vi "Faults and Position data.vi"(8 "error in (no error)":errorcluster, 11 "Controller In":refnum<k24>) -> (0 "error out":errorcluster, 1 "Positions":dbl[](array[numeric]), 2 "Faults":string[](array[string]), 3 "Controller Out":refnum<k24>)   [LabVIEW 2011]
uses:
  C:/Users/Admin/Desktop/Gantry Code Transfer/source/Code Transfer/Aerotech.A3200.dll
  Aerotech.A3200.dll
  AxisDiagPacket.ctl
panel:
  out "Axes":T1[](array[typedef])
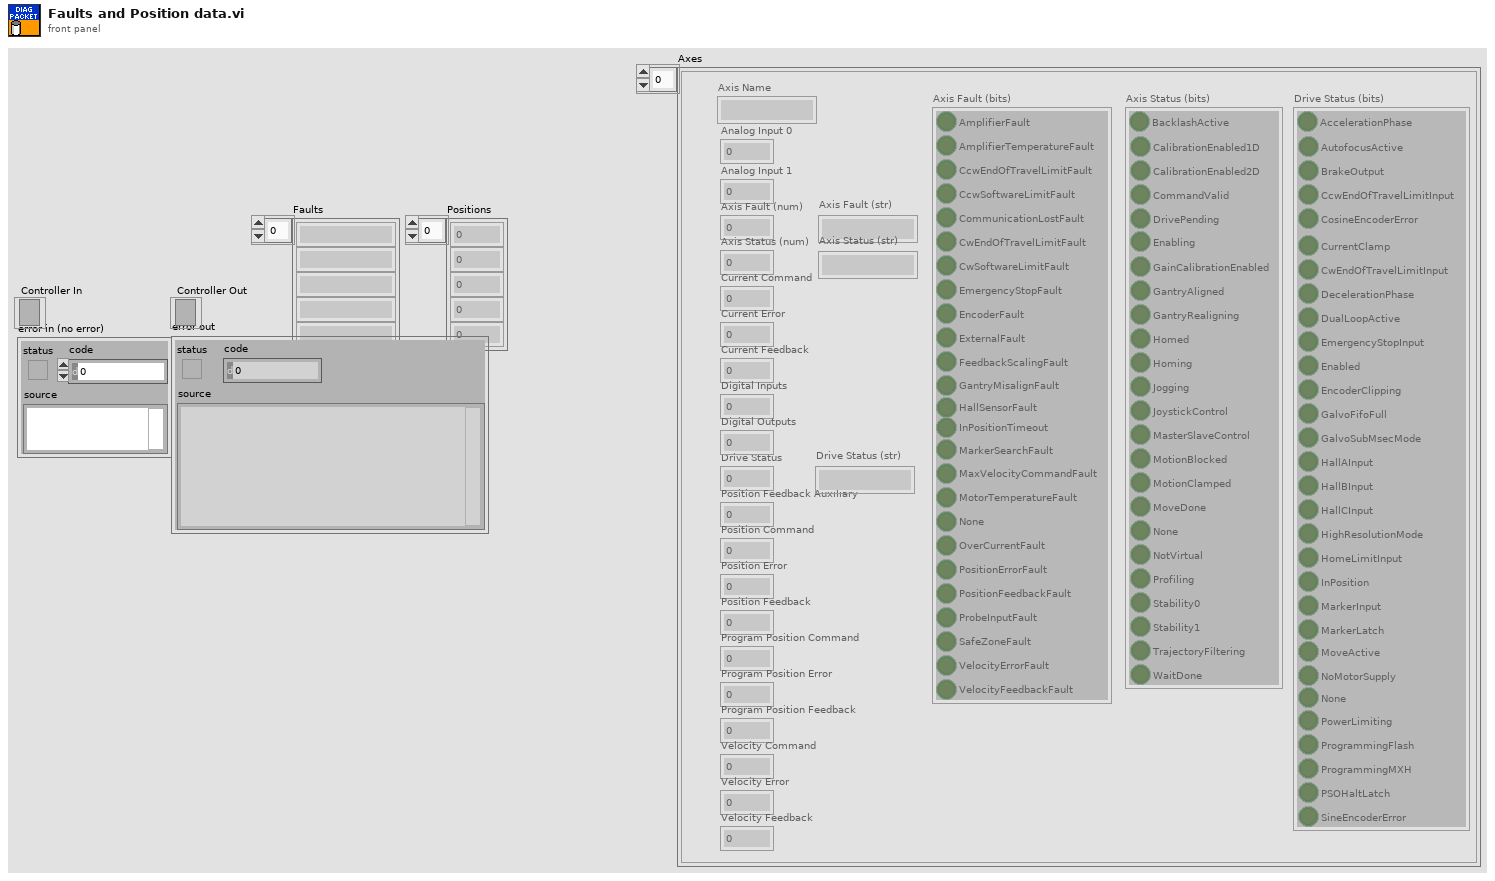
[diagram p1: front panel]
types:
  T1 = typedef "AxisDiagPacket.ctl" = cluster{"Axis Name":string, "Analog Input 0":dbl, "Analog Input 1":dbl, "Axis Fault (num)":i32, "Axis Fault (str)":string, "Axis Fault (bits)":cluster{"AmplifierFault":bool, "AmplifierTemperatureFault":bool, "CcwEndOfTravelLimitFault":bool, "CcwSoftwareLimitFault":bool, "CommunicationLostFault":bool, "CwEndOfTravelLimitFault":bool, "CwSoftwareLimitFault":bool, "EmergencyStopFault":bool, "EncoderFault":bool, "ExternalFault":bool, "FeedbackScalingFault":bool, "GantryMisalignFault ":bool, "HallSensorFault":bool, "InPositionTimeout":bool, "MarkerSearchFault":bool, "MaxVelocityCommandFault":bool, "MotorTemperatureFault":bool, "None":bool, "OverCurrentFault":bool, "PositionErrorFault":bool, "PositionFeedbackFault":bool, "ProbeInputFault":bool, "SafeZoneFault":bool, "VelocityErrorFault":bool, "VelocityFeedbackFault":bool}, "Axis Status (num)":i32, "Axis Status (str)":string, "Axis Status (bits)":cluster{"BacklashActive":bool, "CalibrationEnabled1D":bool, "CalibrationEnabled2D":bool, "CommandValid":bool, "DrivePending":bool, "Enabling":bool, "GainCalibrationEnabled":bool, "GantryAligned":bool, "GantryRealigning":bool, "Homed":bool, "Homing":bool, "Jogging":bool, "JoystickControl":bool, "MasterSlaveControl":bool, "MotionBlocked":bool, "MotionClamped":bool, "MoveDone":bool, "None":bool, "NotVirtual":bool, "Profiling":bool, "Stability0":bool, "Stability1":bool, "TrajectoryFiltering":bool, "WaitDone":bool}, "Current Command":sgl, "Current Error":sgl, "Current Feedback":sgl, "Digital Inputs":i32, "Digital Outputs":i32, "Drive Status":i32, "Drive Status (str)":string, "Drive Status (bits)":cluster{"AccelerationPhase":bool, "AutofocusActive":bool, "BrakeOutput":bool, "CcwEndOfTravelLimitInput":bool, "CosineEncoderError":bool, "CurrentClamp":bool, "CwEndOfTravelLimitInput":bool, "DecelerationPhase":bool, "DualLoopActive":bool, "EmergencyStopInput":bool, "Enabled":bool, "EncoderClipping":bool, "GalvoFifoFull":bool, "GalvoSubMsecMode":bool, "HallAInput":bool, "HallBInput":bool, "HallCInput":bool, "HighResolutionMode":bool, "HomeLimitInput":bool, "InPosition":bool, "MarkerInput":bool, "MarkerLatch":bool, "MoveActive":bool, "NoMotorSupply":bool, "None":bool, "PowerLimiting":bool, "ProgrammingFlash":bool, "ProgrammingMXH":bool, "PSOHaltLatch":bool, "SineEncoderError":bool}, "Position Feedback Auxiliary":dbl, "Position Command":dbl, "Position Error":dbl, "Position Feedback":dbl, "Program Position Command":dbl, "Program Position Error":dbl, "Program Position Feedback":dbl, "Velocity Command":dbl, "Velocity Error":dbl, "Velocity Feedback":dbl}
  T2 = typedef "ControllerDiagPacket.ctl" = cluster{"Number of Diag Packets":i32, "Axes":T1[], "error":errorcluster}
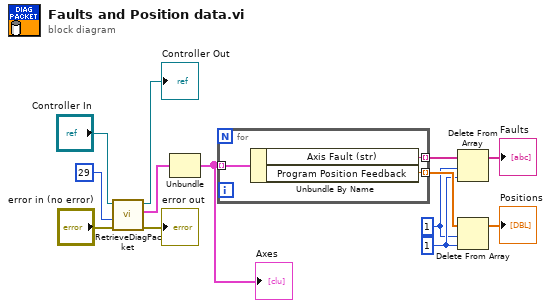
[diagram p0: block diagram]
diagram:
  w1 = 1 ("length")
  w2 = 1 ("index")
  n1 = call "RetrieveDiagPacket.vi"("error in (no error)"="error in (no error)", "axisMask"=29, "Controller In"="Controller In") -> ("error out"=→"error out":errorcluster, "ControllerDiagPacket"=w12:T2, "Controller Out"=→"Controller Out":refnum<k24>)  [unwired: 6 in]
  n2 = Unbundle(w12) -> ("Axes"=w11:T1[])  [unwired: 2 out]
  "Axes" <- w11
  n3 = for {
    tunnel: w11 -> [w16] mode=indexing
    tunnel: [w15] -> w6 mode=indexing
    tunnel: [w14] -> w3 mode=indexing
    n4 = Unbundle By Name(w16) -> ("Axis Fault (str)"=w15:string, "Program Position Feedback"=w14:dbl)
  }
  n5 = Delete From Array(array=w6, length=w1, index=w2) -> (array with subset deleted=→"Faults":string[])  [unwired: 1 out]
  n6 = Delete From Array(array=w3, length=w1, index=w2) -> (array with subset deleted=→"Positions":dbl[])  [unwired: 1 out]
